vi "UHR-Fleezers Control (host) - 11.1.vi"() -> ()   [LabVIEW 2012] (continued)
  in  "Limit Min (MHz)":dbl=10.0 caption="Min (MHz)"
  in  "Limit Max (MHz)":dbl=16.0 caption="Max (MHz)"
  in  "Limits Enable":bool=TRUE caption="Enable"
  out "AI labels":string[](array[string])=["T1 Y", "T1 X", "T1 Sum", "T2 Y", "T2 X", "T2 Sum", "T1 FB X", "T1 FB Sum", "T2 FB X", "T2 FB Sum", "PSD Y", "PSD X", "PSD Y Sum"]
  in  "Save Trap Pos. Data":bool=TRUE
  in  "Lower Ch. Cap.":bool
  in  "Top 3 Harvard Syringe Pump Serial Port":refnum<visa-resource-name>="Top3Harvard"
  # "After"
  # "During"
  # "Trap On?"
  # "BD Flow ON?"
  # "Samp Flow ON?"
  # "Trap Trig. Fl.?"
  # "Zero It"
  # "Floor it\n(e.g., hp unwinding)"
  # "1"
  # "2"
  # "Fl. Down"
  # "Fl. Up"
  # "Bead sep"
  # "Trap Display:"
  # "APD Display:"
  # "DAQ"
  # "Trap Manipulation"
  # "Data Saving"
  # "Bead Calibration"
  # "Bottom Pump (#1)"
  # "Central Sample Channels"
  # "Top Pump (#3)"
  # "Rate param is ul/h\nVolume param is ul"
  # "Chemyx Pump 2"
  # "Units: \n1 = ml/m\n2 = ml/h\n3 = ul/m\n4 = ul/h"
  # "X"
  # "Y"
  # "Oscillate Set 1 freq. (debugging)"
  # "BD 1"
  # "BD 2"
  # "AOD Raster Scan"
  # "Approx. trap separations"
  # "X"
  # "Y"
  # "FPGA\nreading"
  # "DMA\ntransfer"
  # "APD Gates"
  # "APD 2"
  # "APD 1"
  # "X"
  # "2D"
  # "Y"
  # "1D"
  # "Green Laser Interlacing"
  # "Green FB Measurement"
  # "Digital Gate"
  # "Current Analog Control"
  # "Total AI Rates (NOT rates/trap)"
  # "(Samples/trap x Trap Sets)"
  # "(Samples/channel x\n8 if averaging (8 channels)\n4 if no averaging)"
  # "Trap 1"
  # "Trap 2"
  # "Flour./Trap 3"
  # "External Video Window"
  # "MCL Position Debugging"
  # "Temporary Control Storage\n(these used to be somewhere else, still want to keep them)"
  # "Y"
  # "X"
  # "Trap Position Difference Limits"
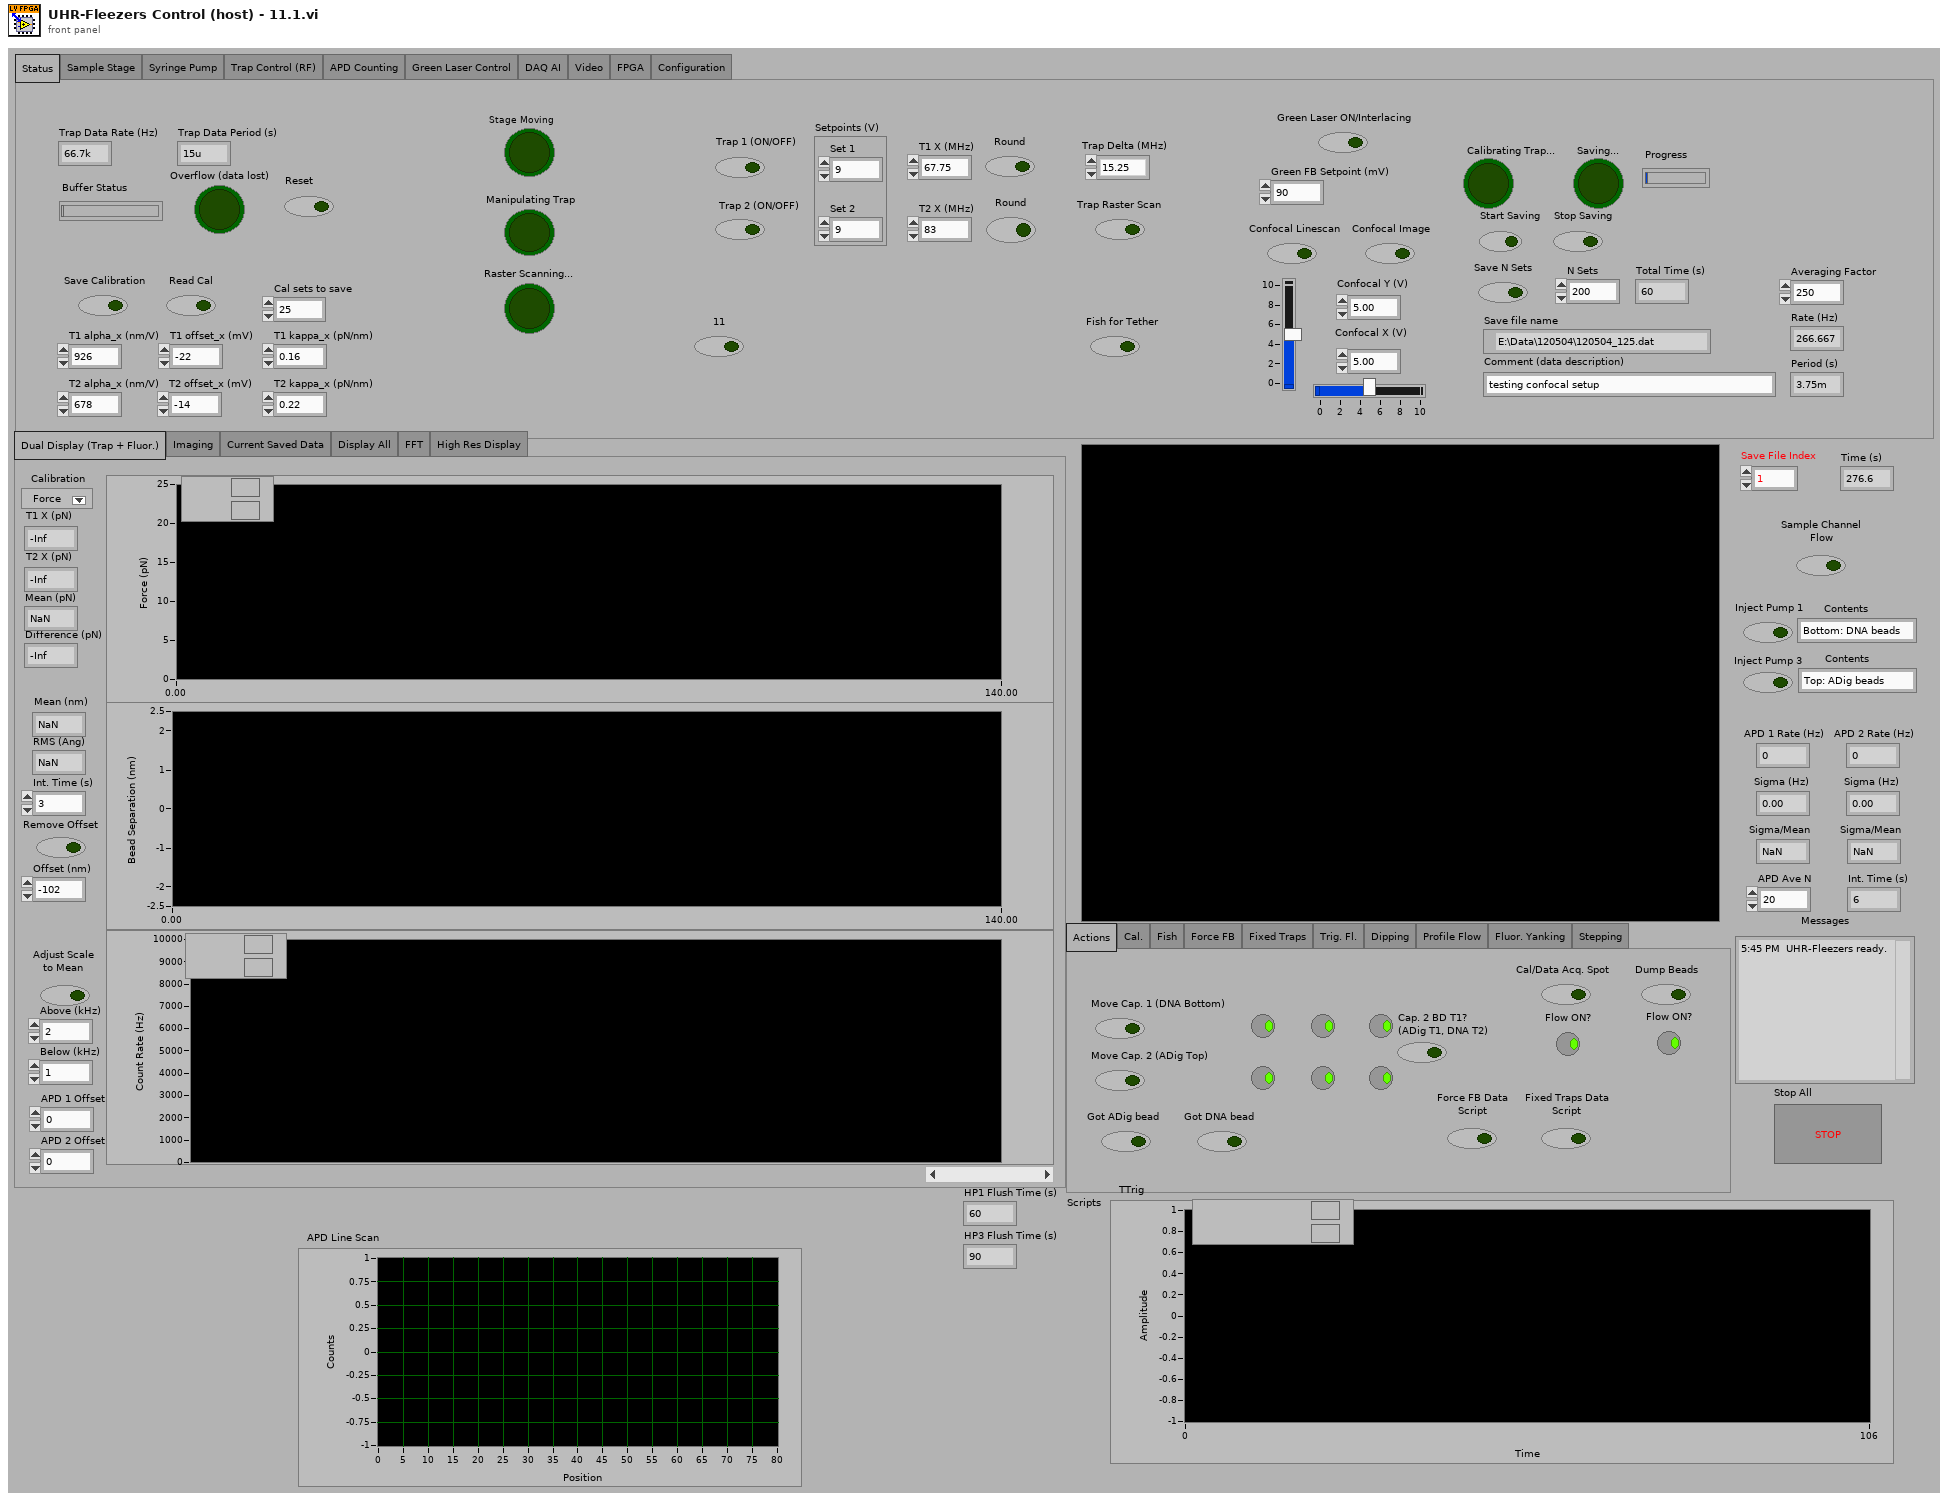
[diagram p1: front panel]
types:
  T1 = enum32{"Actions", "Cal.", "Fish", "Force FB", "Fixed Traps", "Trig. Fl.", "Dipping", "Profile Flow", "Fluor. Yanking", "Stepping"}
  T2 = typedef "IMAQ Image.ctl" = refnum<image>
  T3 = enum32{"Dual Display (Trap + Fluor.)", "Imaging", "Current Saved Data", "Display All", "FFT", "High Res Display"}
  T4 = enum32{"Status", "Sample Stage", "Syringe Pump", "Trap Control (RF)", "APD Counting", "Green Laser Control", "DAQ AI", "Video", "FPGA", "Configuration"}
  T5 = cluster{"Pump 1":cluster{"Diameter (mm)":dbl, "Units":dbl, "Volume":dbl, "Rate":dbl}, "Pump 2":cluster{"Diameter (mm)":dbl, "Units":dbl, "Volume":dbl, "Rate":dbl}, "Pump 3":cluster{"Diameter (mm)":dbl, "Units":dbl, "Volume":dbl, "Rate":dbl}}
  T6 = enum32{"IR Laser Interlacing (Direct RF Board Control Method)", "AOD Raster Scan", "Feedback on Trap Intensity", "Feedback on Trap Position"}
  T7 = typedef "LVPoint32TypeDef.ctl" = cluster{"Horizontal":i32, "Vertical":i32}
  T8 = cluster{"Scan Range AOD (nm) 2":dbl, "Step Size AOD (nm) 2":dbl, "Scan Speed AOD (nm/s) 2":dbl, "Number of scans (AOD) 2":u16, "Label":string}[]
  T9 = cluster{"Set 1":cluster{"proportional gain (Kc)":i16, "integral gain (Kc*Ts/Ti)":i16, "derivative gain (Kc*Td/Ts)":i16}, "Set 2":cluster{"proportional gain (Kc)":i16, "integral gain (Kc*Ts/Ti)":i16, "derivative gain (Kc*Td/Ts)":i16}}
  T10 = cluster{"Trap 1":fxp<+/-,16,1>, "Trap 2":fxp<+/-,16,1>}
  T11 = cluster{"proportional gain (Kc)":fxp<+/-,16,8>, "integral gain (Kc*Ts/Ti)":fxp<+/-,16,8>, "derivative gain (Kc*Td/Ts)":fxp<+/-,16,8>}
  T12 = cluster{"output high":fxp<+/-,16,1>, "output low":fxp<+/-,16,1>}
  T13 = cluster{"Set 1":fxp<+/-,16,1>, "Set 2":fxp<+/-,16,1>}
  T14 = cluster{"proportional gain (Kc)":i16, "integral gain (Kc*Ts/Ti)":i16, "derivative gain (Kc*Td/Ts)":i16}
  T15 = cluster{"Set 1":bool, "Set 2":bool, "Set 3":bool}
  T16 = typedef "LVMinMaxIncTypeDef.ctl" = cluster{"Minimum":dbl, "Maximum":dbl, "Increment":dbl}
  T17 = typedef "Image Type" = u32
  T18 = typedef "nirio_resource_hc.ctl" = tag
  T19 = typedef "openfpgaref.8.6.ctl" = refnum<k20>
  T20 = cluster{"New Image":T2, "New Image":T2, "New Image":T2, "New Image":T2}
  T21 = typedef "XDNodeRunTimeDep.lvlib/timing_clust.ctl" = cluster{"Expected End [f-1]":u64, "Actual End [f-1]":u64, "Finished Late? [f-1]":bool, "Expected End [i-1]":u64, "Actual End [i-1]":u64, "Finished Late? [i-1]":bool, "Expected Start [i]":u64, "Actual Start [i]":u64, "Expected Start [f]":u64, "Actual Start [f]":u64, "Source Name":string, "Structure Name":string, "Period":i64, "Deadline":i64, "Offset":i64, "Start":i64, "Priority":i32, "Timeout":i32, "Mode":T22, "Wakeup Reason":T23, "Error":errorcluster, "Source Type":string, "Secondary Source Type":string, "Global End Time":u64, "Global Start Time":u64, "Frame Duration":u64, "Iteration Duration":u64, "Assigned CPU":i32, "I/O Scan Engine Mode":u32}
  T22 = typedef "XDNodeRunTimeDep.lvlib/nitl_modes.ctl" = enum32{"No Change", "Process missed periods, maintain original phase", "Discard missed periods, maintain original phase", "Process missed periods, ignore original phase", "Discard missed periods, ignore original phase"}
  T23 = typedef "XDNodeRunTimeDep.lvlib/wakeup.ctl" = enum32{"Normal", "Aborted", "Asynchronous wakeup", "Timing source error", "Timed loop error", "Timeout"}
  T24 = cluster{"Left":i32, "Top":i32, "Width":u32, "Height":u32}
  T25 = cluster{cluster{"Left":i32, "Top":i32, "Width":u32, "Height":u32}}[]
  T26 = enum32{"setting", "request", "request control", "info", "statistics", "system settings", "I/O sub system", "HRT control", "camera descriptions", "device specific data", "event sub system settings", "event sub system results", "image memory manager"}
  T27 = typedef "AviRefnum.ctl" = refnum<k1>
  T28 = typedef "imagedata.ctl" = cluster{"image type":i32, "image depth":i32, "image":u8[], "mask":u8[], "colors":u32[], "Rectangle":cluster{"left":i16, "top":i16, "right":i16, "bottom":i16}}
  T29 = enum32{"Normal Display", "Dual Display (APD)", "FFT", "High Res Display"}
  T30 = cluster{"Origin Pixel":cluster{"X":sgl, "Y":sgl}, "Angle Relative to Horizontal (deg)":sgl, "Axis Reference":u32}
  T31 = typedef "Simple Grid Descriptor" = cluster{"X Step":sgl, "Y Step":sgl, "Unit":T32}
  T32 = typedef "Image Unit" = enum32{"Undefined", "Angström", "Micrometer", "Millimeter", "Centimeter", "Meter", "Kilometer", "Microinch", "Inch", "Feet", "Nautical miles", "Standard miles", "Steps"}
  T33 = cluster{"averaging mode":u16, "weighting mode":u16, "number of averages":u32}
  T34 = cluster{"dB On (F)":bool, "unwrap phase (F)":bool, "convert to degree (F)":bool}
  T35 = enum16{"open", "replace", "create", "open or create", "replace or create", "replace or create with confirmation"}
  T36 = enum16{"big-endian, network order", "native, host order", "little-endian"}
  T37 = cluster{string, string, string, string, string, string, string, string}
  T38 = cluster{string, string, string, string, string, string, string, string, string, string, string, string}
  T39 = cluster{string, string, string, string, string, string, string, string, string, string, string, string, string}
  T40 = cluster{string, string, string, string, string, string, string, string, string, string, string, string, string, string}
  T41 = cluster{"BD 1 Frequency 1 (MHz)":dbl, "BD 1 Frequency 2 (MHz)":dbl}
  T42 = cluster{"f0":dbl, "df":dbl, "magnitude":dbl[]}[][]
  T43 = cluster{"Green FB Ch 0":i16, "Green FB Ch 1":i16, "Green FB Ch 2":i16}
  T44 = cluster{"Green FB Ch 0":dbl, "Green FB Ch 1":dbl, "Green FB Ch 2":dbl}
  T45 = cluster{"Scan Range AOD (nm) 2":dbl, "Step Size AOD (nm) 2":dbl, "Scan Speed AOD (nm/s) 2":dbl, "Number of scans (AOD) 2":u16, "Label":string}
  T46 = cluster{"[0]":dbl, "[1]":dbl, "[2]":dbl, "[3]":dbl, "[4]":dbl, "[5]":dbl}
  T47 = cluster{"Diameter (mm)":dbl, "Units":dbl, "Volume":dbl, "Rate":dbl}
diagram:
  w12 = u16 20 items=["1.0"=10, "1.5"=15, "2.0"=20] ("stop bits (10: 1 bit)")
  w15 = u16 20 items=["1.0"=10, "1.5"=15, "2.0"=20] ("stop bits (10: 1 bit)")
  w72 = u16 20 items=["1.0"=10, "1.5"=15, "2.0"=20] ("stop bits (10: 1 bit)")
  w79 = T17 2 items=["Grayscale (U8)", "Grayscale (I16)", "Grayscale (SGL)", "Complex (CSG)", "RGB (U32)", "HSL (U32)", "RGB (U64)", "Grayscale (U16)"] ("Image Type")
  w142 = cluster{"output high":i16, "output low":i16} {"output high"=3000, "output low"=0} ("FB output range 1")
  w213 = 10.0 ("y")
  w212 = 32767.0 ("y")
  w228 = 6.0  # clock mult.
  w229 = 49152000.0  # TCXO frequ.
  # "Bottom 1 Harvard"
  # "Top 3 Harvard"
  # "Center Harvard"
  # "Bottom 1 Harvard"
  # "Top 3 Harvard"
  # "Center Harvard"
  n1 = Build Array("DIO count 1 (ticks)", "DIO count 2 (ticks)", "DIO count 3 (ticks)") -> (w129:u32[])
  n2 = local read "AO1"() -> (w207:dbl)
  n3 = local read "AO2"() -> (w206:dbl)
  n4 = local read "Scan Increment (MHz)"() -> (w224:dbl)
  n5 = local read "Continuous MCL Scanning"() -> (w194:bool)
  n6 = local read "Fast Scan Dir"() -> (w193:bool)
  n7 = local read "Number of scans (MCL)"() -> (w195:u64)
  n8 = property on="AI Count (ticks)" class="DigNum (strict)"("Val(Sgnl)"="AI Count (ticks)") -> ()  [unwired: 2 in, 2 out]
  n9 = Multiply(x=w207, y=w212) -> (x*y=w209:dbl)
  n10 = Multiply(x=w206, y=w212) -> (x*y=w211:dbl)
  n11 = Divide(x=w209, y=w213) -> (x/y=w208:dbl)
  n12 = Divide(x=w211, y=w213) -> (x/y=w210:dbl)
  n13 = To Word Integer(number=w208) -> (16bit integer=w205:i16)
  n14 = To Word Integer(number=w210) -> (16bit integer=w204:i16)
  n15 = Not(x=w193) -> (.not. x?=w188:bool)
  n16 = local read "Cycles/step (MCL)"() -> (w196:u64)
  n17 = Multiply(x=w224, y=1000.0) -> (x*y=w231:dbl)
  n18 = local read "Scan steps (MCL)"() -> (w197:u64)
  n19 = local write "Trap Pos FIFO Timeout"(u16 0 ("Trap Pos FIFO Timeout")) -> ()
  n20 = local read "Desired Scan Incr (V)"() -> (w199:dbl)
  n21 = Scale By Power Of 2(n=48, x=w231) -> (x*2^n=w232:dbl)
  n22 = Multiply(x=w229, y=w228) -> (x*y=w227:dbl)
  n23 = Divide(x=w232, y=w227) -> (x/y=w226:dbl)
  n24 = local read "Setpoints (V)"() -> (w245:cluster{"Set 1":dbl, "Set 2":dbl})
  n25 = To Quad Integer(1:w226) -> (0:w223:i64)
  n26 = Divide(x=40000000.0, y="AI Count (ticks)") -> (x/y=w184:dbl)
  n27 = Multiply(x=w199, y=32767.0) -> (x*y=w201:dbl)
  n28 = local read "Number Interlace Sets"() -> (w122:u8)
  n29 = Split 1D Array(array=w129, index=w122) -> (first subarray=w131:u32[])  [unwired: 1 out]
  n30 = Add Array Elements(numeric array=w131) -> (sum=w130:u32)
  n31 = local read "# Samples/channel"() -> (w216:u32)
  n32 = local read "Number of F/B Scans (AOD)"() -> (w217:u16)
  n33 = local read "Not-Interlacing Set"() -> (w121:enum32{"Set 1", "Set 2", "Set 3"})
  n34 = To Unsigned Byte Integer(number=w121) -> (unsigned 8bit integer=w127:u8)
  n35 = Index Array(array=w129, index=w127) -> (element=w128:u32)
  n36 = local read "Feedback On/Off"() -> (w248:cluster{"Set 1":bool, "Set 2":bool})
  n37 = local read "PID Gains"() -> (w240:T9)
  n38 = local read "Scan steps (AOD)"() -> (w222:u64)
  n39 = local read "All FB On/Off"() -> (w249:bool)
  n40 = local read "Cycles/step (AOD)"() -> (w221:u64)
  n41 = local write "AI rate (Hz)"(w184) -> ()
  n42 = Divide(x=w201, y=10.0) -> (x/y=w200:dbl)
  n43 = Multiply(x=w222, y=w221) -> (x*y=w220:u64)
  n44 = Multiply(x=3276.7, y=w245) -> (x*y=w244:cluster{"Set 1":dbl, "Set 2":dbl})
  n45 = xnode "FPGA Open VI Reference"("resource name"=T18 "750kHzDAQ") -> ("FPGA VI Reference Out"=w237:T19, "error out"=w236:errorcluster)  [unwired: 1 in]
  n46 = To Word Integer(number=w200) -> (16bit integer=w198:i16)
  n47 = Multiply(x=w220, y=u64 2) -> (x*y=w218:u64)
  n48 = local read "Sets to FIFO (Traps)"() -> (w252:T15)
  n49 = Divide(x=w184, y="FPGA Ave.") -> (x/y=w185:dbl)
  n50 = To Word Integer(number=w244) -> (16bit integer=w243:cluster{"Set 1":i16, "Set 2":i16})
  n51 = Unbundle By Name(w240) -> ("Set 1"=w239:T14, "Set 2"=w238:T14)
  n52 = Multiply(x=w218, y=w217) -> (x*y=w215:u64)
  n53 = local write "Ave. Rate (Hz)"(w185) -> ()
  n54 = Divide(x=w215, y=w216) -> (x/y=w214:dbl)
  n55 = Unbundle By Name(w243) -> ("Set 1"=w242:i16, "Set 2"=w241:i16)
  n56 = local read "2D or 1D Scan"() -> (w143:bool)
  n57 = local write "Data points/scans"(w215) -> ()
  n58 = local read "Scan BD"() -> (w233:bool)
  n59 = And(x=w248, y=w249) -> (x .and. y?=w247:cluster{"Set 1":bool, "Set 2":bool})
  n60 = local write "Data points/scan (f/b)"(w218) -> ()
  n61 = Reciprocal(x=w185) -> (1/x=w186:dbl)
  n62 = local read "N Acq Sets (Traps + Fl.)"() -> (w177:i16)
  n63 = local write "N sets should be saved"(w214) -> ()
  n64 = xnode "Invoke Method"("FPGA VI Reference In"=w237, "error in"=w236) -> ("FPGA VI Reference Out"=w141:T19, "error out"=w151:errorcluster)
  n65 = Unbundle By Name(w247) -> ("Set 1"=w251:bool, "Set 2"=w250:bool)
  n66 = local read "Interlace"() -> (w123:bool)
  n67 = Select(t=w130, s=w123, f=w128) -> (s? t:f=w120:u32)
  n68 = local write "Update Count (MCL)"(w120) -> ()
  n69 = local write "Total Counts (ticks)"(w120) -> ()
  n70 = local write "Ave. Period (s)"(w186) -> ()
  n71 = property on="2D or 1D Scan" class="Bool (strict)"("Val(Sgnl)"=w143) -> ()  [unwired: 2 in, 2 out]
  n72 = local read "GI Frequency, OFF count"() -> (w44:u32)
  n73 = local read "GI Frequency, ON count"() -> (w35:u32)
  n74 = local read "APD Gate OFF Count"() -> (w41:u32)
  n75 = local read "APD Gate ON Count"() -> (w37:u32)
  n76 = xnode "Read/Write Control"("FPGA VI Reference In"=w140, "error in"=w151, "ai count"="AI Count (ticks)", "Interlace ON/OFF"=w123, "Number Interlace Cycles"=w122, "AI1 Sets to FIFO"=w252, "FB On/Off Set 1"=w251, "FB On/Off Set 2"=w250, "Interlace Off Parameters"=w121, "FB Setpoint Set 1"=w242, "FB Setpoint Set 2"=w241, "FB Gains Set 1"=w239, "FB Gains Set 2"=w238, "FB output range 1"=w142, "FB output range 2"=w142, "Cycles per step"=w221, "Scan BD"=w233, "Number of scans"=w217, "Scan steps"=w222, "Scan freq.  increment"=w223, "AO1"=w205, "AO2"=w204, "Scan freq.  increment (MCL)"=w198, "Scan steps (MCL)"=w197, "Cycles per step (MCL)"=w196, "Number of scans (MCL)"=w195, "MCL count"=w120, "Cont. Scan (MCL)"=w194, "MCL Scan Axis"=w188, "1D or 2D Scan?"=w143, "N of AI1 Int Acq Sets"=w177, "Freq or Amp switch first"="Freq or Amp switch first", "Freq switch delay"="Freq switch delay", "Amp switch delay"="Amp switch delay", "Swap F1 and F2"="Swap F1 and F2", "APD to FIFO"=FALSE, "DIO count 1 (ticks)"="DIO count 1 (ticks)", "DIO count 2 (ticks)"="DIO count 2 (ticks)", "DIO count 3 (ticks)"="DIO count 3 (ticks)") -> ("FPGA VI Reference Out"=w48:T19, "error out"=w46:errorcluster)  [unwired: 1 in]
  n77 = local read "On one out of X cycles"() -> (w43:u32)
  n78 = local read "APD Integration Time (s)"() -> (w27:dbl)
  n79 = local read "DMA Update Period (s)"() -> (w26:dbl)
  n80 = Add(x=w37, y=w41) -> (x+y=w39:u32)
  n81 = Add(x=w35, y=w44) -> (x+y=w42:u32)
  n82 = local read "Green Laser ON/Interlacing"() -> (w118:bool)
  n83 = local read "Green laser mode"() -> (w119:enum32{"Laser ON", "Laser OFF", "Interlace"})
  n84 = Multiply(x=w39, y=w43) -> (x*y=w40:u32)
  n85 = Multiply(x=w43, y=w42) -> (x*y=w34:u32)
  n86 = Reciprocal(x=w27) -> (1/x=w24:dbl)
  n87 = Multiply(x=w27, y=40000000.0) -> (x*y=w23:dbl)
  n88 = Divide(x=w26, y=w27) -> (x/y=w29:dbl)
  n89 = Multiply(x="Current When FB OFF (%)", y=655.35) -> (x*y=w106:dbl)
  n90 = local read "Invert APD Gate"() -> (w33:bool)
  n91 = Multiply(x="Green FB Setpoint (mV)", y=3.2767) -> (x*y=w103:dbl)
  n92 = local read "APD Gate"() -> (w32:enum32{"ON", "OFF", "Interlace"})
  n93 = Subtract(x=w40, y=w37) -> (x-y=w38:u32)
  n94 = local write "Green FB Count"(w34) -> ()
  n95 = local write "APD Acq Rate (Hz)"(w24) -> ()
  n96 = To Unsigned Long Integer(number=w23) -> (unsigned 32bit integer=w21:u32)
  n97 = Multiply(x=2.0, y=w29) -> (x*y=w28:dbl)
  n98 = local read "Invert GI"() -> (w115:bool)
  n99 = To Unsigned Word Integer(number=w106) -> (unsigned 16bit integer=w104:u16)
  n100 = Subtract(x=w34, y=w35) -> (x-y=w36:u32)
  n101 = local write "APD Samples/FIFO Acq."(w29) -> ()
  n102 = To Word Integer(number=w103) -> (16bit integer=w101:i16)
  n103 = local write "APD Elements/DMA read"(w28) -> ()
  n104 = case shown="False" w118 {
    tunnel: w119 -> [_ w278]
    tunnel: [enum32{"Laser ON", "Laser OFF", "Interlace"}."Laser OFF" ("Green laser mode") w278] -> w114
    frame False {
    }
    frame True {
    }
  }
  n105 = local write "APD Int. Count"(w21) -> ()
  n106 = local read "Trap Pos. AI1 X Pre-scale"() -> (w58:u16)
  n107 = local read "Trap Pos FB Monitor\nT1 or T2"() -> (w65:bool)
  n108 = local read "Trap Pos FB Int Count"() -> (w52:u16)
  n109 = local read "APD 1 AO Mult."() -> (w31:i16)
  n110 = local read "Trap Pos FB Negate Action"() -> (w64:bool)
  n111 = local read "APD 2 AO Mult."() -> (w30:i16)
  n112 = local read "Trap Pos. FB Offset Factor"() -> (w63:i64)
  n113 = local read "Trap Pos. FB Mult Factor"() -> (w62:i64)
  n114 = local read "Differential FB?"() -> (w18:bool)
  n115 = local read "Neg. TTrig FPGA"() -> (w20:bool)
  n116 = local read "Trap Pos. FB Gains"() -> (w60:T11)
  n117 = local read "Trap Pos. FB Range"() -> (w61:T12)
  n118 = xnode "Read/Write Control"("FPGA VI Reference In"=w48, "error in"=w46, "Invert APD Gate"=w33, "APD Gate ON Count"=w37, "APD Gate OFF Count"=w38, "APD Acq Rate Count"=w21, "APD Gate Operating Mode"=w32, "APD 1 AO scale factor"=w31, "APD 2 AO scale factor"=w30, "Green interlace ON count"=w35, "Green interlace OFF count"=w36, "Green interlace ON count 2"=w35, "Green interlace OFF count 2"=w36, "Green FB Count"=w34) -> ("FPGA VI Reference Out"=w47:T19, "error out"=w45:errorcluster)
  n119 = xnode "Read/Write Control"("FPGA VI Reference In"=w47, "error in"=w45, "Invert GI 2"=w115, "Operating Mode 2"=w114, "Green FB Gains"="Green FB Gains", "Green FB Setpoint"=w101, "Green FB On/Off"="Green FB On/Off", "Current Out"=w104, "Green int current ON count adj"="Green int current ON count adj", "Operating Mode"=w114, "Invert GI"=w115, "Trap Pos FB Monitor T1 or T2"=w65, "Trap Pos FB Negate Action"=w64, "Trap Pos. FB Offset Factor"=w63, "Trap Pos. FB Mult Factor"=w62, "Trap Pos. FB Range"=w61, "Trap Pos. FB Gains"=w60, "Force feedback"=FALSE, "AI1 X Scale"=w58, "Trap Pos to FIFO"=TRUE, "Trap Pos FB Int Count"=w52, "TTrig Negate Pos"=w20, "FB Trig Integrate"="FB Trig Integrate", "Diff FB Measurement?"=w18, "Negate Diff?"="Negate Diff?") -> ("FPGA VI Reference Out"=w116:T19, "error out"=w117:errorcluster)
  n120 = xnode "Invoke Method"("FPGA VI Reference In"=w116, "error in"=w117, "Depth"="Trap AI FIFO Depth") -> ("FPGA VI Reference Out"=w68:T19, "error out"=w67:errorcluster)
  n121 = xnode "Invoke Method"("FPGA VI Reference In"=w68, "error in"=w67, "Depth"="Trap Position FIFO Depth") -> ("FPGA VI Reference Out"=w54:T19, "error out"=w53:errorcluster)
  n122 = flat-sequence {
    tunnel: w141 -> [w283]
    tunnel: [w283] -> w140
    tunnel: [w282] -> w139
    tunnel: [w281] -> w138
    tunnel: [w279] -> w136
    tunnel: [w280] -> w137
    frame #0 {
      w280 = T16 {"Minimum"=0.0, "Maximum"=40.0, "Increment"=1.0} ("Min Max Inc")
      w279 = T16 {"Minimum"=0.0, "Maximum"=50.0, "Increment"=1.0} ("Data Entry Limits")
      w282 = T16 {"Minimum"=60.0, "Maximum"=90.0, "Increment"=1.0} ("Min Max Inc")
      w281 = T16 {"Minimum"=0.0, "Maximum"=50.0, "Increment"=1.0} ("Data Entry Limits")
      n123 = property on="BD 2 Frequency 1 (MHz)" class="DigNum (strict)"("Data Range"=w280) -> ()  [unwired: 2 in, 2 out]
      n124 = property on="BD 2 Frequency 3 (MHz)" class="DigNum (strict)"("Data Range"=w280) -> ()  [unwired: 2 in, 2 out]
      n125 = property on="BD 2 Frequency 2 (MHz)" class="DigNum (strict)"("Data Range"=w280) -> ()  [unwired: 2 in, 2 out]
      n126 = property on="BD 1 Frequency 1 (MHz)" class="DigNum (strict)"("Data Range"=w282) -> ()  [unwired: 2 in, 2 out]
      n127 = property on="BD 1 Frequency 2 (MHz)" class="DigNum (strict)"("Data Range"=w282) -> ()  [unwired: 2 in, 2 out]
      n128 = property on="BD 1 Frequency 3 (MHz)" class="DigNum (strict)"("Data Range"=w282) -> ()  [unwired: 2 in, 2 out]
      n129 = property on="BD 2 Amplitude 1 (%)" class="DigNum (strict)"("Data Range"=w279) -> ()  [unwired: 2 in, 2 out]
      n130 = property on="BD 2 Amplitude 2 (%)" class="DigNum (strict)"("Data Range"=w279) -> ()  [unwired: 2 in, 2 out]
      n131 = property on="BD 2 Amplitude 3 (%)" class="DigNum (strict)"("Data Range"=w279) -> ()  [unwired: 2 in, 2 out]
      n132 = property on="BD 1 Amplitude 3 (%)" class="DigNum (strict)"("Data Range"=w281) -> ()  [unwired: 2 in, 2 out]
      n133 = property on="BD 1 Amplitude 2 (%)" class="DigNum (strict)"("Data Range"=w281) -> ()  [unwired: 2 in, 2 out]
      n134 = property on="BD 1 Amplitude 1 (%)" class="DigNum (strict)"("Data Range"=w281) -> ()  [unwired: 2 in, 2 out]
      "X RF Frequency Limits (MHz)" <- w282
      "X RF Amplitude Limits (%)" <- w281
      "Y RF Amplitude Limits (%)" <- w279
      "Y RF Frequency Limits (MHz)" <- w280
    }
  }
  n135 = xnode "Invoke Method"("FPGA VI Reference In"=w54, "error in"=w53) -> ("FPGA VI Reference Out"=w150:T19, "error out"=w149:errorcluster)  [unwired: 1 in]
  n136 = flat-sequence "Initial FPGA Loop Relative Phase Adjustment" {
    tunnel: "Initial Phase Adjustment (AI1)" -> [w294]
    tunnel: "Initial Phase Adjustment (GI)" -> [w293]
    tunnel: w150 -> [w292]
    tunnel: w149 -> [w291]
    tunnel: "Initial Phase Adj. (MCL)" -> [w290]
    tunnel: [w295] -> w159
    tunnel: [w289] -> w155
    tunnel: "Initial Phase Adjustment (APD Acq)" -> [w288]
    tunnel: "Initial Phase Adjustment (APD 1 Gate)" -> [w287]
    tunnel: "Initial Phase Adjustment (Green FB)" -> [w286]
    tunnel: "Initial Phase Adjustment (GI) 2" -> [w285]
    tunnel: "Initial Phase Adjustment (APD 2 Gate)" -> [w284]
    tunnel: w159 -> [w297]
    tunnel: [w298] -> w156
    tunnel: w155 -> [w298]
    tunnel: [w297] -> w154
    tunnel: w156 -> [w301]
    tunnel: w154 -> [w300]
    tunnel: [w303] -> w153
    tunnel: [w302] -> w152
    tunnel: [w305] -> w157
    tunnel: [w306] -> w158
    tunnel: w153 -> [w306]
    tunnel: w152 -> [w305]
    frame #0 {
      n137 = xnode "Read/Write Control"("FPGA VI Reference In"=w292, "error in"=w291, "Phase count adjustment"=w294, "Phase count adjustment (GI)"=w293, "Phase count adjustment (MCL)"=w290, "Phase Count Adjustment (APD Acq)"=w288, "Phase count adjustment (APD 1 Gate)"=w287, "Phase count adjustment (APD 2 Gate)"=w284, "Phase count adjustment (Green FB)"=w286, "Phase count adjustment (GI) 2"=w285) -> ("FPGA VI Reference Out"=w289:T19, "error out"=w295:errorcluster)
    }
    frame #1 {
      n138 = Wait (ms)(milliseconds to wait=u32 100) -> ()  [unwired: 1 out]
    }
    frame #2 {
      w299 = TRUE
      n139 = xnode "Read/Write Control"("FPGA VI Reference In"=w301, "error in"=w300, "+ phase"=w299, "+ phase (GI)"=w299, "+ phase (MCL)"=w299, "+ phase (APD Acq)"=w299, "+ phase (APD 1 Gate)"=w299, "+ phase (APD 2 Gate)"=w299, "+ phase (Green FB)"=w299, "+ phase (GI) 2"=w299) -> ("FPGA VI Reference Out"=w302:T19, "error out"=w303:errorcluster)
    }
    frame #3 {
      n140 = Wait (ms)(milliseconds to wait=u32 100) -> ()  [unwired: 1 out]
    }
  }
  n141 = local read "Phase adj. (Green FB)"() -> (w132:i16)
  n142 = local read "Phase adj. (GI) 2"() -> (w107:i16)
  n143 = local read "Phase adjust (MCL)"() -> (w189:i16)
  n144 = local read "Phase adj. (AI1)"() -> (w191:i16)
  n145 = local read "Phase adj. (GI)"() -> (w190:i16)
  n146 = xnode "Read/Write Control"("FPGA VI Reference In"=w157, "error in"=w158, "Phase count adjustment"=w191, "Phase count adjustment (GI)"=w190, "Phase count adjustment (MCL)"=w189, "Phase Count Adjustment (APD Acq)"="Phase Adj. (APD Acq)", "Phase count adjustment (APD 1 Gate)"="Phase Adj. (APD 1 Gate)", "Phase count adjustment (APD 2 Gate)"="Phase Adj. (APD 2 Gate)", "Phase count adjustment (Green FB)"=w132, "Phase count adjustment (GI) 2"=w107) -> ("FPGA VI Reference Out"=w93:T19, "error out"=w166:errorcluster)
  n147 = call "Initialize RF boards - interlace 3.vi"("error in"=w166, "FPGA VI Reference In"=w93) -> ("error out"=w164:errorcluster, "FPGA VI Reference Out"=w165:T19)
  n148 = call "set RF board frequency - interlace.vi"("Board 2 Frequency Limits"=w137, "Board 1 Frequency Limits"=w139, "error in"=w164, "FPGA VI Reference In"=w165, "Board 2 Frequency 3 (MHz)"="BD 2 Frequency 3 (MHz)", "Board 1 Frequency 3 (MHz)"="BD 1 Frequency 3 (MHz)", "Board 2 Frequency 2 (MHz)"="BD 2 Frequency 2 (MHz)", "Board 2 Frequency 1 (MHz)"="BD 2 Frequency 1 (MHz)", "Board 1 Frequency 2 (MHz)"="BD 1 Frequency 2 (MHz)", "Board 1 Frequency 1  (MHz)"="BD 1 Frequency 1 (MHz)") -> ("error out"=w267:errorcluster, "FPGA VI Reference Out"=w268:T19)
  n149 = call "set RF board amplitude - interlace.vi"("Board 2 Amplitude Limits"=w136, "Board 1 Amplitude Limits"=w138, "error in"=w267, "FPGA VI Reference In"=w268, "Board 2 Amplitude 3 (%)"="BD 2 Amplitude 3 (%)", "Board 1 Amplitude 3 (%)"="BD 1 Amplitude 3 (%)", "Board 2 Amplitude 2 (%)"="BD 2 Amplitude 2 (%)", "Board 2 Amplitude 1 (%)"="BD 2 Amplitude 1 (%)", "Board 1 Amplitude 2 (%)"="BD 1 Amplitude 2 (%)", "Board 1 Amplitude 1 (%)"="BD 1 Amplitude 1 (%)") -> ("error out"=w255:errorcluster, "FPGA VI Reference Out"=w256:T19)
  n150 = flat-sequence {
    tunnel: w256 -> [w316]
    tunnel: w255 -> [w315]
    tunnel: [w314] -> w260
    tunnel: [w313] -> w259
    tunnel: [w320] -> w258
    tunnel: w260 -> [w320]
    tunnel: [w319] -> w257
    tunnel: w259 -> [w319]
    tunnel: w258 -> [w329]
    tunnel: w257 -> [w328]
    tunnel: [w327] -> w6
    tunnel: [w326] -> w55
    frame #0 {
      w307 = FALSE ("Retract Pump 3")
      n151 = local read "Trap 1 (ON/OFF)"() -> (w308:bool)
      n152 = xnode "Read/Write Control"("FPGA VI Reference In"=w316, "error in"=w315, "Direct RF Box  Communication"=FALSE) -> ("FPGA VI Reference Out"=w314:T19, "error out"=w313:errorcluster)
      n153 = local write "Saving..."(FALSE ("Saving Data")) -> ()
      n154 = local write "Stop All"(FALSE ("Stop All")) -> ()
      n155 = local write "Retract Pump 1"(w307) -> ()
      n156 = local write "Retract Pump 3"(w307) -> ()
      n157 = local write "Index"(1.0 ("Index")) -> ()
      n158 = property on="Trap 1 ON" class="Bool (strict)"("Value"=w308) -> ()  [unwired: 2 in, 2 out]
      "Manipulating Trap" <- FALSE ("Manipulating Trap")
    }
    frame #1 {
      n159 = local read "Trap 2 (ON/OFF)"() -> (w318:bool)
      n160 = Wait (ms)(milliseconds to wait=u32 10) -> ()  [unwired: 1 out]
      n161 = property on="Trap 2 ON" class="Bool (strict)"("Val(Sgnl)"=w318) -> ()  [unwired: 2 in, 2 out]
    }
    frame #2 {
      n162 = local read "Scan Range (nm)"() -> (w322:dbl)
      n163 = xnode "Read/Write Control"("FPGA VI Reference In"=w329, "error in"=w328, "FPGA Controls  RF Box"=TRUE ("Direct RF Box  Communication")) -> ("FPGA VI Reference Out"=w327:T19, "error out"=w326:errorcluster)
      n164 = call "Update messages.vi"("Message to add"="UHR-Fleezers ready.", "Old message string"="") -> ("New message string"=w325:string)
      n165 = local write "Messages"(w325) -> ()
      n166 = property on="Scan Range (nm)" class="DigNum (strict)"("Val(Sgnl)"=w322) -> ()  [unwired: 2 in, 2 out]
    }
  }
  n167 = Subtract(x="BD 1 Frequency 1 (MHz)", y="BD 1 Frequency 2 (MHz)") -> (x-y=w176:dbl)
  n168 = Subtract(x="BD 2 Frequency 1 (MHz)", y="BD 2 Frequency 2 (MHz)") -> (x-y=w175:dbl)
  n169 = Square(x=w175) -> (x^2=w173:dbl)
  n170 = Square(x=w176) -> (x^2=w174:dbl)
  n171 = Add(x=w174, y=w173) -> (x+y=w172:dbl)
  n172 = Square Root(x=w172) -> (sqrt(x)=w171:dbl)
  n173 = local write "Trap Delta (MHz)"(w171) -> ()
  n174 = call "IMAQ Create"("Image Name"="APD 1 Image", "Image Type"=w79) -> ("New Image"=w78:T2)  [unwired: 3 in, 1 out]
  n175 = call "IMAQ Create"("Image Name"="APD 2 Image", "Image Type"=w79) -> ("New Image"=w77:T2)  [unwired: 3 in, 1 out]
  n176 = call "IMAQ Create"("Image Name"="Det. X Image", "Image Type"=w79) -> ("New Image"=w76:T2)  [unwired: 3 in, 1 out]
  n177 = call "IMAQ Create"("Image Name"="Det. Y Image", "Image Type"=w79) -> ("New Image"=w75:T2)  [unwired: 3 in, 1 out]
  n178 = Bundle("New Image"=w78, "New Image"=w77, "New Image"=w76, "New Image"=w75) -> (w74:T20)  [unwired: 1 in]
  n179 = call-poly "VISA Configure Serial Port"("VISA resource name"="Bottom  1 Harvard Syringe Pump Serial Port", "baud rate (9600)"=u32 115200, "stop bits (10: 1 bit)"=w12) -> ("VISA resource name out"=w8:refnum<visa-resource-name>, "error out"=w7:errorcluster)  [unwired: 4 in, 7 out]
  n180 = call-poly "VISA Configure Serial Port"("VISA resource name"="Top 3 Harvard Syringe Pump Serial Port", "baud rate (9600)"=u32 115200, "stop bits (10: 1 bit)"=w15) -> ("VISA resource name out"=w10:refnum<visa-resource-name>, "error out"=w9:errorcluster)  [unwired: 4 in, 7 out]
  n181 = call-poly "VISA Configure Serial Port"("VISA resource name"="Sample Chamber Stage Serial Port") -> ("VISA resource name out"=w88:refnum<visa-resource-name>, "error out"=w89:errorcluster)  [unwired: 5 in, 8 out]
  "Stage Control Serial Error" <- w89
  n182 = call-poly "VISA Configure Serial Port"("VISA resource name"="Center Harvard Syringe Pump Serial Port", "baud rate (9600)"=u32 115200, "stop bits (10: 1 bit)"=w72) -> ("VISA resource name out"=w69:refnum<visa-resource-name>, "error out"=w70:errorcluster)  [unwired: 4 in, 7 out]
  n183 = node-c288() -> (w99:T21)  [unwired: 4 out]
  n184 = node-c288() -> (w84:T21)  [unwired: 4 in]
  n185 = disable-structure shown="Disabled" {
    disable-tunnel: [w332 _] -> w235
    disable-tunnel: w6 -> [w331 _]
    frame Disabled {
      n186 = node-c288() -> (w334:T21)  [unwired: 4 out]
      n187 = timed-loop "Rough control of MCL mirror stage (debugging)" {
        tunnel: w331 -> [w337]
        tunnel: [w336] -> w332
        timing: w334 -> [_]
        timing-out: [_] -> w333
        stop <- w336 stop-if-true
        n188 = node-c288() -> ()  [unwired: 2 out]
        n189 = case shown="1" "MCL Mode" {
          tunnel: w337 -> [_ w340 w387]
          frame 0, Default {
          }
          frame 1 {
            n190 = node-c288() -> (w342:T21)  [unwired: 4 out]
            n191 = timed-loop "Oscillate MCL mirror" {
              timing: w342 -> [_]
              timing-out: [_] -> w341
              tunnel: w340 -> [w381]
              i -> [w380]
              stop <- w343 stop-if-true
              n192 = node-c288() -> (w379:i64)  [unwired: 1 out]
              n193 = Multiply(x="AO1", y=32767.0) -> (x*y=w375:dbl)
              n194 = Multiply(x="AO2", y=32767.0) -> (x*y=w370:dbl)
              n195 = Divide(x=w375, y=10.0) -> (x/y=w376:dbl)
              n196 = Divide(x=w370, y=10.0) -> (x/y=w371:dbl)
              n197 = To Word Integer(number=w376) -> (16bit integer=w368:i16)
              n198 = To Word Integer(number=w371) -> (16bit integer=w367:i16)
              n199 = Divide(x=w379, y=i64 1000) -> (x/y=w350:dbl)
              n200 = Multiply(x=w350, y=w380) -> (x*y=w361:dbl)
              n201 = Multiply(x="Osc. freq. (Hz) 2", y=6.283185307179586) -> (x*y=w362:dbl)
              n202 = Multiply(x=w362, y=w361) -> (x*y=w360:dbl)
              n203 = Sine(x=w360) -> (sin(x)=w359:dbl)
              n204 = Multiply(x=w359, y="Osc. amp. (V)") -> (x*y=w357:dbl)
              n205 = Add(x=w357, y="Osc. center (V)") -> (x+y=w355:dbl)
              n206 = Divide(x=w355, y=10.0) -> (x/y=w353:dbl)
              n207 = Multiply(x=w353, y=32767.0) -> (x*y=w348:dbl)
              n208 = Select(t=w348, s="Scan axis", f=w368) -> (s? t:f=w366:dbl)
              n209 = Select(t=w367, s="Scan axis", f=w348) -> (s? t:f=w365:dbl)
              n210 = local read "MCL Mode"() -> (w347:u16)
              n211 = Not Equal?(x=w347, y=u16 1) -> (x != y?=w344:bool)
              n212 = local read "Stop All"() -> (w345:bool)
              n213 = xnode "Read/Write Control"("FPGA VI Reference In"=w381, "AO1"=w366, "AO2"=w365) -> ()  [unwired: 1 in, 2 out]
              n214 = Compound Arithmetic op=OR(w345, w344) -> (w343:bool)
              n215 = node-c288() -> ()  [unwired: 2 out]
            }
            n216 = node-c288(w341) -> ()  [unwired: 1 out]
          }
          frame 2 {
            n217 = case shown="True" "Start Scan" {
              tunnel: w387 -> [_ w399]
              frame False {
              }
              frame True {
                n218 = Subtract(x="End (V)", y="Begin (V)") -> (x-y=w395:dbl)
                n219 = Decrement(x="N Points") -> (x-1=w394:dbl)
                n220 = Divide(x=w395, y=w394) -> (x/y=w392:dbl)
                n221 = for {
                  N: "N Points" -> [_]
                  tunnel: "Begin (V)" -> [w412]
                  tunnel: w399 -> [w404]
                  tunnel: [w403] -> w398 mode=indexing
                  tunnel: w392 -> [w402]
                  tunnel: [w400] -> w391 mode=indexing
                  i -> [w411]
                  n222 = Multiply(x=w402, y=w411) -> (x*y=w410:dbl)
                  n223 = Add(x=w412, y=w410) -> (x+y=w407:dbl)
                  n224 = local read "Scan axis"() -> (w401:bool)
                  n225 = local read "AO1"() -> (w409:dbl)
                  n226 = local read "AO2"() -> (w408:dbl)
                  n227 = Select(t=w407, s=w401, f=w409) -> (s? t:f=w406:dbl)
                  n228 = Select(t=w408, s=w401, f=w407) -> (s? t:f=w405:dbl)
                  n229 = flat-sequence {
                    tunnel: w406 -> [w416]
                    tunnel: w405 -> [w415]
                    tunnel: w404 -> [w413]
                    tunnel: [w426] -> w403
                    tunnel: [w425] -> w400
                    frame #0 {
                      w419 = 10.0 ("y")
                      w414 = 32767.0 ("y")
                      n230 = Multiply(x=w416, y=w414) -> (x*y=w422:dbl)
                      n231 = Multiply(x=w415, y=w414) -> (x*y=w420:dbl)
                      n232 = Divide(x=w422, y=w419) -> (x/y=w423:dbl)
                      n233 = Divide(x=w420, y=w419) -> (x/y=w421:dbl)
                      n234 = To Word Integer(number=w423) -> (16bit integer=w417:i16)
                      n235 = To Word Integer(number=w421) -> (16bit integer=w418:i16)
                      n236 = xnode "Read/Write Control"("FPGA VI Reference In"=w413, "AO1"=w417, "AO2"=w418) -> ()  [unwired: 1 in, 2 out]
                    }
                    frame #1 {
                      n237 = Wait (ms)(milliseconds to wait="DAQ Delay (ms)") -> ()  [unwired: 1 out]
                    }
                    frame #2 {
                      n238 = local read "Slow mean"() -> (w426:dbl)
                      n239 = local read "Sigma"() -> (w425:dbl)
                    }
                  }
                }
                n240 = Bundle("Begin (V)"="Begin (V)", w392, w398) -> (→"MCL Scan":cluster{"Begin (V)":dbl, dbl, dbl[]})  [unwired: 1 out]
                n241 = Bundle("Begin (V)"="Begin (V)", w392, w391) -> (→"MCL Scan 2":cluster{"Begin (V)":dbl, dbl, dbl[]})  [unwired: 1 out]
              }
            }
          }
        }
        n242 = local read "Stop All"() -> (w336:bool)
        n243 = node-c288() -> ()  [unwired: 2 out]
      }
      n244 = node-c288(w333) -> ()  [unwired: 1 out]
    }
    frame Enabled {
    }
  }
  n245 = node-c288(i64 1 ("Period"), 1 ("Processor")) -> (w180:T21)  [unwired: 2 out]
  n246 = node-c288(2 ("Processor")) -> (w97:T21)  [unwired: 3 out]
  n247 = timed-loop "Mouse control: trap position (AOM deflection), set confocal spot from image" {
    tunnel: [w430] -> w187
    tunnel: w6 -> [w429]
    timing: w99 -> [_]
    timing-out: [_] -> w98
    stop <- w430 stop-if-true
    n248 = node-c288() -> ()  [unwired: 2 out]
    n249 = event shown="[0] \"Pane\": Mouse Down" {
      selector: _ -> [_ _]
      dyn-events: _ -> [_ _]
      timeout: _ -> [_ _]
      tunnel: w429 -> [w433 _]
      event Mouse Down {
        n250 = event-data() -> ("Time"=w435:u32, "Coords"=w434:T7, "Button"=w436:u16)  [unwired: 6 out]
        n251 = case shown="1" w436 {
          tunnel: w435 -> [_ _ w542]
          tunnel: w434 -> [_ w473 w540]
          tunnel: w433 -> [_ _ w538]
          frame 0, Default {
          }
          frame 1 {
            n252 = property on="APD 2" class="ImageControl"() -> ("Displayed Image Position"=w443:cluster{"Left":i32, "Top":i32})  [unwired: 2 in, 2 out]
            n253 = property on="APD 1" class="ImageControl"() -> ("Displayed Image Position"=w472:cluster{"Left":i32, "Top":i32})  [unwired: 2 in, 2 out]
            n254 = property on="Detection Laser X" class="ImageControl"() -> ("Displayed Image Position"=w469:cluster{"Left":i32, "Top":i32})  [unwired: 2 in, 2 out]
            n255 = property on="Detection Laser Y" class="ImageControl"() -> ("Displayed Image Position"=w468:cluster{"Left":i32, "Top":i32})  [unwired: 2 in, 2 out]
            n256 = property on="APD 2" class="ImageControl"() -> ("Displayed Image Size"=w442:cluster{"Width":u32, "Height":u32})  [unwired: 2 in, 2 out]
            n257 = property on="APD 1" class="ImageControl"() -> ("Displayed Image Size"=w470:cluster{"Width":u32, "Height":u32})  [unwired: 2 in, 2 out]
            n258 = property on="Detection Laser X" class="ImageControl"() -> ("Displayed Image Size"=w471:cluster{"Width":u32, "Height":u32})  [unwired: 2 in, 2 out]
            n259 = property on="Detection Laser Y" class="ImageControl"() -> ("Displayed Image Size"=w467:cluster{"Width":u32, "Height":u32})  [unwired: 2 in, 2 out]
            n260 = Unbundle By Name(w442) -> ("Width"=w439:u32, "Height"=w438:u32)
            n261 = Unbundle By Name(w443) -> ("Left"=w441:i32, "Top"=w440:i32)
            n262 = Unbundle By Name(w470) -> ("Width"=w464:u32, "Height"=w463:u32)
            n263 = Unbundle By Name(w471) -> ("Width"=w460:u32, "Height"=w459:u32)
            n264 = Unbundle By Name(w467) -> ("Width"=w456:u32, "Height"=w455:u32)
            n265 = Unbundle By Name(w472) -> ("Left"=w466:i32, "Top"=w465:i32)
            n266 = Unbundle By Name(w469) -> ("Left"=w462:i32, "Top"=w461:i32)
            n267 = Unbundle By Name(w468) -> ("Left"=w458:i32, "Top"=w457:i32)
            n268 = Bundle("Left"=w441, "Top"=w440, "Width"=w439, "Height"=w438) -> (w437:T24)  [unwired: 1 in]
            n269 = Bundle("Left"=w466, "Top"=w465, "Width"=w464, "Height"=w463) -> (w454:T24)  [unwired: 1 in]
            n270 = Bundle("Left"=w462, "Top"=w461, "Width"=w460, "Height"=w459) -> (w453:T24)  [unwired: 1 in]
            n271 = Bundle("Left"=w458, "Top"=w457, "Width"=w456, "Height"=w455) -> (w452:T24)  [unwired: 1 in]
            n272 = Build Cluster Array(w437, w454, w453, w452) -> (w451:T25)
            n273 = for {
              tunnel: w473 -> [w484]
              tunnel: w451 -> [w485] mode=indexing
              shift-right: [w482] -> w449
              shift-left: TRUE -> [w483]
              shift-right: [w481] -> w447
              shift-left: _ -> [w477]
              shift-right: [w480] -> w446
              shift-left: _ -> [w476]
              shift-right: [w479] -> w445
              shift-left: _ -> [w475]
              shift-right: [w478] -> w444
              shift-left: _ -> [w474]
              n274 = case shown="True" w483 {
                selector: w483 -> [w490 _]
                tunnel: w485 -> [_ w499]
                tunnel: w484 -> [_ w497]
                tunnel: [w490 w495] -> w482
                tunnel: [w489 w494] -> w481
                tunnel: [w488 w493] -> w480
                tunnel: [w487 w492] -> w479
                tunnel: [w486 w491] -> w478
                tunnel: w477 -> [w489 _]
                tunnel: w476 -> [w488 _]
                tunnel: w475 -> [w487 _]
                tunnel: w474 -> [w486 _]
                frame False {
                }
                frame True {
                  n275 = Unbundle(w499) -> (w498:T24)
                  n276 = call "isclickinwindow.vi"("Image Param"=w498, "Point32"=w497) -> ("4 Y"=w491:i32, "3 Height"=w492:i32, "2 X"=w493:i32, "1 Width"=w494:i32, "In image?"=w496:bool)  [unwired: 1 in]
                  n277 = Not(x=w496) -> (.not. x?=w495:bool)
                }
              }
            }
            n278 = Not(x=w449) -> (.not. x?=w448:bool)
            n279 = case shown="True" w448 {
              tunnel: w446 -> [_ w513]
              tunnel: w444 -> [_ w512]
              tunnel: w447 -> [_ w511]
              tunnel: w445 -> [_ w510]
              frame False {
              }
              frame True {
                w500 = FALSE ("Get Point")
                n280 = local read "Scan lines (y)"() -> (w515:u64)
                n281 = disable-structure shown="Disabled" {
                  frame Disabled {
                  }
                  frame Enabled {
                  }
                }
                n282 = local read "Actual MCL Inc (V)"() -> (w509:dbl)
                n283 = local read "Scan steps (MCL)"() -> (w514:u64)
                n284 = Divide "Y Pix/step"(x=w510, y=w515) -> (x/y=w522:dbl)
                n285 = Divide "Y V/pix"(x=w509, y=w522) -> (x/y=w521:dbl)
                n286 = Divide "Y half step offset"(x=w509, y=2.0) -> (x/y=w523:dbl)
                n287 = Divide "X pix/step"(x=w511, y=w514) -> (x/y=w520:dbl)
                n288 = Negate(x=w523) -> (-x=w524:dbl)
                n289 = local read "Initial Y"() -> (w530:dbl)
